vi "LVCAM Destroy Self.vi"(11 "LVCAM Destroy Self in":refnum<class "LVCAM Destroy Self.lvclass">) -> (0 "error out":errorcluster, 1 "Destroyed Self?":bool, 3 "LVCAM Destroy Self out":refnum<class "LVCAM Destroy Self.lvclass">)   [LabVIEW 2021, in "LVCAM Destroy Self.lvlib" / "LVCAM Destroy Self.lvclass"]
uses:
  LVCAM Destroy Self.lvclass
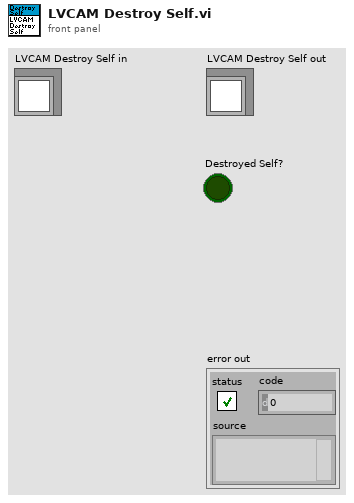
[diagram p1: front panel]
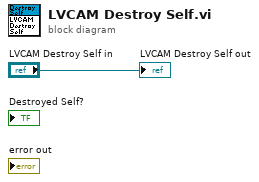
[diagram p0: block diagram]
diagram:
  "LVCAM Destroy Self out" <- "LVCAM Destroy Self in"
